vi "Write channels.vi"(8 "error in (no error)":errorcluster, 10 "channels":refnum<class "TBM channel.lvclass">[](array[class]), 11 "bin datalogger configuration in":refnum<class "Binary datalogger configuration.lvclass">) -> (0 "error out":errorcluster, 3 "bin datalogger configuration out":refnum<class "Binary datalogger configuration.lvclass">)   [LabVIEW 2013, in "Binary datalogger configuration.lvclass"]
uses:
  Binary datalogger configuration.lvclass
  <vilib>/NI/Tag Bus Module Framework/channel/TBM channel.lvclass
  Binary datalogger configuration.lvclass/Binary datalogger configuration.ctl
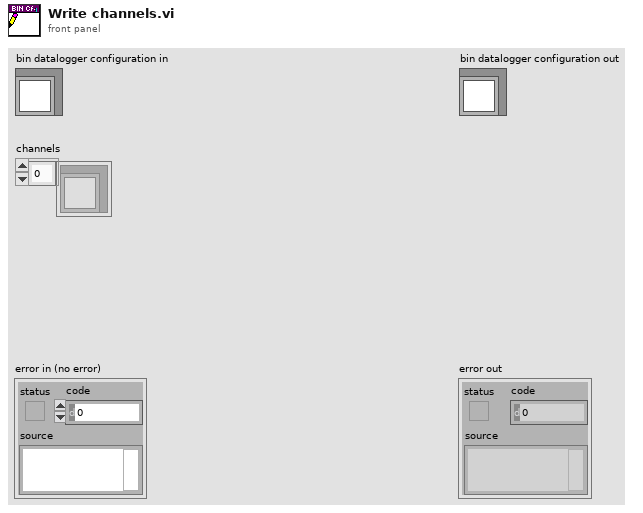
[diagram p1: front panel]
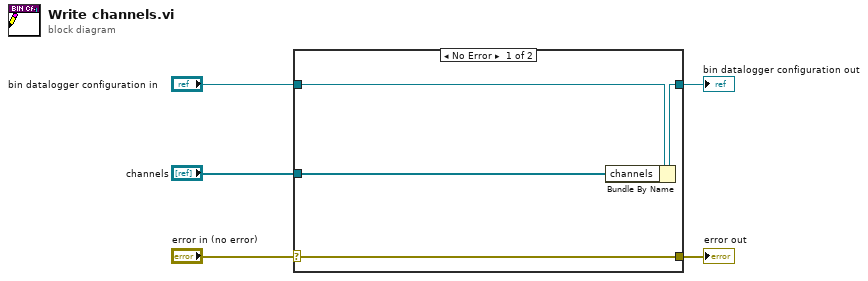
[diagram p0: block diagram]
diagram:
  n1 = case shown="No Error" "error in (no error)" {
    selector: "error in (no error)" -> [w9 w10]
    tunnel: [w9 w10] -> w4
    tunnel: [w7 w11] -> w2
    tunnel: "bin datalogger configuration in" -> [w8 w11]
    tunnel: "channels" -> [w6 _]
    frame No Error {
      n2 = Bundle By Name(cluster=w8, "channels"=w6) -> (w7:refnum<class "Binary datalogger configuration.lvclass">)
    }
    frame Error {
    }
  }
  "error out" <- w4
  "bin datalogger configuration out" <- w2
